vi "dfd_CIC_Interpolator.vi"(10 "input valid":bool=TRUE, 11 "input data":bool[](array[boolean])) -> (0 "ready for input":bool, 2 "output valid":bool, 3 "output data":bool[](array[boolean]))   [LabVIEW 2017]
uses:
  <vilib>/rvi/FXPMathLib/basic elements/FxpDiscreteDelay/XNode/nifxpmath_DiscreteDelay.xnode
  <vilib>/rvi/FXPMathLib/basic elements/FxpAddSub/XNode/nifxpmath_AddSub.xnode
  <vilib>/rvi/FXPMathLib/sim/FxpSim.dll
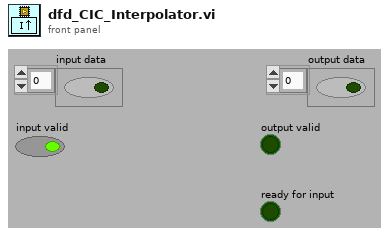
[diagram p1: front panel]
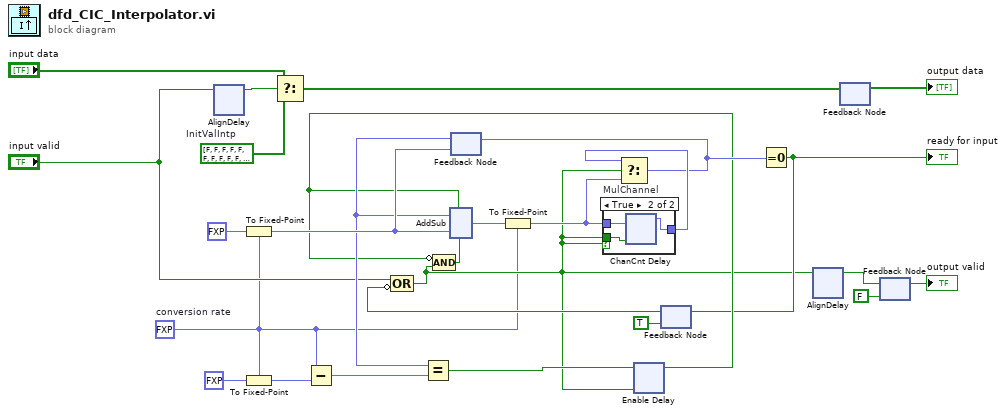
[diagram p0: block diagram]
diagram:
  w1 = fxp<+,2,2> 2.0  # conversion rate
  w24 = bool[] [FALSE, FALSE, FALSE, FALSE, FALSE, FALSE, FALSE, FALSE, FALSE, FALSE, FALSE, FALSE, FALSE, FALSE, FALSE, FALSE, FALSE, FALSE, FALSE, FALSE, FALSE, FALSE, FALSE, FALSE, FALSE, FALSE, FALSE, FALSE, FALSE, FALSE, FALSE, FALSE, FALSE, FALSE, FALSE, FALSE, FALSE, FALSE, FALSE, FALSE, FALSE, FALSE, FALSE, FALSE, FALSE, FALSE, FALSE, FALSE, FALSE, FALSE, FALSE, FALSE, FALSE, FALSE, FALSE, FALSE, FALSE, FALSE, FALSE, FALSE, FALSE, FALSE, FALSE, FALSE, FALSE, FALSE, FALSE, FALSE, FALSE, FALSE, FALSE, FALSE, FALSE, FALSE, FALSE, FALSE, FALSE, FALSE, FALSE, FALSE, FALSE, FALSE, FALSE, FALSE, FALSE, FALSE, FALSE, FALSE, FALSE, FALSE, FALSE, FALSE, FALSE, FALSE, FALSE, FALSE, FALSE, FALSE, FALSE, FALSE, FALSE, FALSE, FALSE, FALSE, FALSE, FALSE, FALSE, FALSE, FALSE, FALSE, FALSE, FALSE, FALSE, FALSE, FALSE, FALSE, FALSE, FALSE, FALSE, FALSE, FALSE, FALSE, FALSE, FALSE, FALSE, FALSE, FALSE, FALSE, FALSE, FALSE, FALSE, FALSE, FALSE, FALSE, FALSE, FALSE, FALSE, FALSE, FALSE, FALSE, FALSE, FALSE, FALSE, FALSE, FALSE, FALSE, FALSE, FALSE, FALSE, FALSE, FALSE, FALSE, FALSE, FALSE, FALSE, FALSE, FALSE, FALSE, FALSE, FALSE, FALSE, FALSE, FALSE, FALSE, FALSE, FALSE, FALSE, FALSE, FALSE, FALSE, FALSE, FALSE, FALSE, FALSE, FALSE, FALSE, FALSE, FALSE, FALSE, FALSE, FALSE, FALSE, FALSE, FALSE, FALSE, FALSE, FALSE, FALSE, FALSE, FALSE, FALSE, FALSE]  # InitValIntp
  n1 = xnode "AlignDelay"("D"="input valid") -> ("Q"=w17:bool)
  n2 = To Fixed-Point(fixed-point type=w1, number=fxp<+,2,2> 0.0 ("fixed-point")) -> (fixed-point=w26:fxp<+,2,2>)
  n3 = To Fixed-Point(fixed-point type=w1, number=fxp<+,2,2> 2.0 ("fixed-point")) -> (fixed-point=w27:fxp<+,2,2>)
  n4 = Select(t="input data", s=w17, f=w24) -> (s? t:f=w10:bool[])
  n5 = Subtract(x=w1, y=w27) -> (x-y=w21:fxp<+/-,3,3>)
  n6 = feedback #1(w26) -> (w22:fxp<+,2,2>)
  n7 = Equal?(x=w22, y=w21) -> (x = y?=w14:bool)
  n8 = feedback #2(TRUE) -> (w19:bool)
  n9 = Compound Arithmetic op=OR("input valid", invert w19) -> (w4:bool)
  n10 = xnode "Enable Delay"("D"=w14, "enable"=w4) -> ("Q"=w13:bool)
  n11 = Compound Arithmetic op=AND(invert w13, w4) -> (w23:bool)
  n12 = xnode ("AddSub")("x"=w22, "y"=w26, "carry-in"=w23, "use zero instead of x"=w13) -> ("s"=w16:fxp<+,2,2>)  [unwired: 1 out]
  n13 = To Fixed-Point(fixed-point type=w1, number=w16) -> (fixed-point=w15:fxp<+,2,2>)
  n14 = case "MulChannel" shown="True" w4 {
    tunnel: [w28 w31] -> w25
    tunnel: w15 -> [w28 w30]
    tunnel: w4 -> [_ w29]
    frame False {
    }
    frame True {
      n15 = xnode ("ChanCnt Delay")("D"=w30, "enable"=w29) -> ("Q"=w31:fxp<+,2,2>)
    }
  }
  n16 = Select(t=w25, s=w4, f=w15) -> (s? t:f=w20:fxp<+,2,2>)
  n17 = feedback-in #1(w20) -> ()
  n18 = Equal To 0?(x=w20) -> (x = 0?=w8:bool)
  "ready for input" <- w8
  n19 = feedback-in #2(w8) -> ()
  n20 = xnode "AlignDelay"("D"=w4) -> ("Q"=w7:bool)
  n21 = feedback-in #3(w10) -> ()
  n22 = feedback #3() -> (→"output data":bool[])  [unwired: 1 out]
  n23 = feedback-in #4(w7) -> ()
  n24 = feedback #4(FALSE ("Q")) -> (→"output valid":bool)
